vi "Main.vi"() -> ()   [LabVIEW 2012]
uses:
  MeasureDialogButton.ctl
  SourceDialogButton.ctl
  TriggerDialogButton.ctl
  DUTDisplayData.ctl
  DUTDialogButton.ctl
  LogDialogButton.ctl
  Setup.ctl
  DUTConfiguration.ctl
  driver/Public/Controls/SMUSense.ctl
  LogConfiguration.ctl
  LogStartConfiguration.ctl
  LogStartTriggerType.ctl
  LogDigitalIOTriggerEdge.ctl
  LogRolloverConfiguration.ctl
  LogRolloverTriggerType.ctl
  LogStopConfiguration.ctl
  LogStopTriggerType.ctl
  TriggerConfiguration.ctl
  TriggerInputConfiguration.ctl
  TriggerInputType.ctl
  driver/Public/Controls/TriggerMode.ctl
  TriggerOutputConfiguration.ctl
  TriggerOutputType.ctl
  SourceConfiguration.ctl
  SourceFunction.ctl
  MeasureConfiguration.ctl
  driver/Public/Controls/SMU.ctl
  UIActionQueueElement.ctl
  UIAction.ctl
  HardwareActionQueueElement.ctl
  HardwareAction.ctl
  HardwareAbortGlobalAction.ctl
  LogActionQueueElement.ctl
  LogAction.ctl
  driver/Keithley-2602.lvlib
  libs/LV-Utilities/LV-Utilities.lvlib
panel:
  in  "LIVE":bool
  in  "SYSTEM":bool
  out "Tab Control":enum32{"SYSTEM", "LIVE"}(tab)
  out "Digital IO Port":bool[](array[boolean])
  out "Setup File":path
  in  "RESET":bool
  in  "SAVE":bool
  in  "OPEN":bool
  in  "LOG START":bool
  out "Log Running?":bool
  in  "Hardware START":bool
  out "Hardware Running?":bool
  in  "SHOW LOG DIALOG":T1
  in  "SHOW DUT DIALOG":T2
  in  "SHOW SOURCE DIALOG":T3
  in  "SHOW TRIGGER DIALOG":T4
  in  "SHOW MEASURE DIALOG":T5
  out "System SMU B DUT Display Data":T6[](array[typedef]) {"Resistance (Ohm)" format="%_4p"; "Current (A)" format="%_4p"; "Voltage (V)" format="%_4p"}
  out "System SMU A DUT Display Data":T6[](array[typedef]) {"Resistance (Ohm)" format="%_4p"; "Current (A)" format="%_4p"; "Voltage (V)" format="%_4p"}
  out "Log File":path
  out "Live SMU Chart":dbl(graph)
  in  "Live Measure Value":enum16{"Voltage", "Current", "Resistance"}(ring)
  in  "Live SMU":enum16{"A", "B"}(ring)
  in  "Live DUT":u32=1 min=1 step=1
  out "Live SMU Value":dbl format="%_4p"
  out "Live SMU Units":enum16{"V", "A", "Ohm"}(ring)
  in  "CHART SMU DATA RESET":bool
  in  "DONE":bool
  # "DIGITAL IO"
  # "1"
  # "2"
  # "3"
  # "4"
  # "5"
  # "6"
  # "7"
  # "8"
  # "9"
  # "10"
  # "11"
  # "12"
  # "13"
  # "14"
  # "SETUP"
  # "LOG"
  # "RUN"
  # "SMU B"
  # "SMU A"
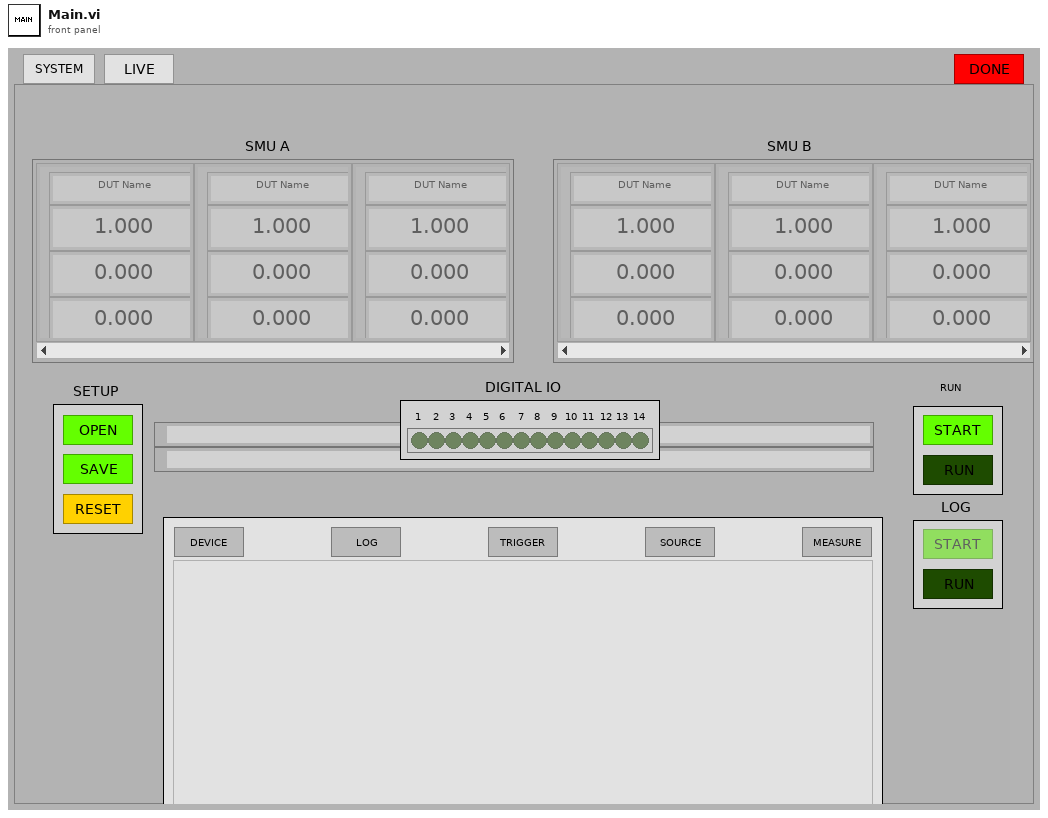
[diagram p1: front panel]
types:
  T1 = typedef "LogDialogButton.ctl" = bool
  T2 = typedef "DUTDialogButton.ctl" = bool
  T3 = typedef "SourceDialogButton.ctl" = bool
  T4 = typedef "TriggerDialogButton.ctl" = bool
  T5 = typedef "MeasureDialogButton.ctl" = bool
  T6 = typedef "DUTDisplayData.ctl" = cluster{"Name":string, "Voltage (V)":dbl, "Current (A)":dbl, "Resistance (Ohm)":dbl}
  T7 = typedef "Setup.ctl" = cluster{"DUT":T8, "Log":T10, "Trigger":T18, "Sources":T24[], "Measures":T26[]}
  T8 = typedef "DUTConfiguration.ctl" = cluster{"Count":u32, "Wirings":T9[], "Names":string[][]}
  T9 = typedef "Keithley-2602.lvlib/SMUSense.ctl" = enum16{"Local (2-wire)", "Remote (4-wire)", "Calibration"}
  T10 = typedef "LogConfiguration.ctl" = cluster{"Start":T11, "Rollover":T14, "Stop":T16}
  T11 = typedef "LogStartConfiguration.ctl" = cluster{"Trigger Type":T12, "Timer (sec)":dbl, "Digital IO Line":u8, "Digital IO Edge":T13}
  T12 = typedef "LogStartTriggerType.ctl" = enum16{"Immediate", "User", "Timer", "Digital IO"}
  T13 = typedef "LogDigitalIOTriggerEdge.ctl" = enum16{"Rising", "Falling"}
  T14 = typedef "LogRolloverConfiguration.ctl" = cluster{"Trigger Type":T15, "Timer (sec)":dbl, "File Size (MB)":u32, "Digital IO Line":u8, "Digital IO Edge":T13}
  T15 = typedef "LogRolloverTriggerType.ctl" = enum16{"None", "Timer", "File Size", "Digital IO"}
  T16 = typedef "LogStopConfiguration.ctl" = cluster{"Trigger Type":T17, "Timer (sec)":dbl, "File Size (MB)":u32, "Digital IO Line":u8, "Digital IO Edge":T13}
  T17 = typedef "LogStopTriggerType.ctl" = enum16{"None", "User", "Timer", "File Size", "Digital IO"}
  T18 = typedef "TriggerConfiguration.ctl" = cluster{"Input":T19, "Output":T22}
  T19 = typedef "TriggerInputConfiguration.ctl" = cluster{"Type":T20, "Timeout (ms)":u32, "Delay (ms)":u32, "Digital IO Line (1-14)":u8, "Digital IO Mode":T21}
  T20 = typedef "TriggerInputType.ctl" = enum16{"None", "Digital IO", "Bus"}
  T21 = typedef "Keithley-2602.lvlib/TriggerMode.ctl" = enum16{"Falling", "Rising", "Either", "Synchronous"}
  T22 = typedef "TriggerOutputConfiguration.ctl" = cluster{"Type":T23, "Delay (ms)":u32, "Digital IO Line (1-14)":u8, "Digital IO Mode":T21, "Digital IO Pulse Width (sec)":dbl}
  T23 = typedef "TriggerOutputType.ctl" = enum16{"None", "Digital IO", "Bus"}
  T24 = typedef "SourceConfiguration.ctl" = cluster{"Enabled?":bool, "Function":T25, "Level (V or A)":dbl, "Autorange Enabled?":bool, "High Limit (V or A)":dbl, "Low Limit (V or A)":dbl}
  T25 = typedef "SourceFunction.ctl" = enum16{"Voltage", "Current"}
  T26 = typedef "MeasureConfiguration.ctl" = cluster{"Enabled?":bool, "Count":u8, "Interval (sec)":dbl, "Voltage Auto Range Enabled?":bool, "Voltage High Limit (V or A)":dbl, "Voltage Low Limit (V or A)":dbl, "Current Auto Range Enabled?":bool, "Current High Limit (V or A)":dbl, "Current Low Limit (V or A)":dbl}
  T27 = typedef "ExecutableConfiguration.ctl" = cluster{"GPIB ID":u8, "GPIB Board":u8, "Default Data Folder":path, "Default Setup Folder":path}
  T28 = typedef "DataStructures.ctl" = cluster{"Display Data":refnum<notifier>, "Log Data":refnum<queue>}
  T29 = typedef "ActionQueues.ctl" = cluster{"UI Action":refnum<queue>, "Hardware Action":refnum<queue>, "Log Action":refnum<queue>}
  T30 = typedef "Keithley-2602.lvlib/SMU.ctl" = enum16{"A", "B"}
  T31 = enum8{"Enabled", "Disabled", "Disabled and Grayed Out"}
  T32 = typedef "UIActionQueueElement.ctl" = cluster{"Action":T33, "Data":variant}
  T33 = typedef "UIAction.ctl" = enum16{"Initialize", "Configure Trigger", "Configure Measure", "Configure Source", "Configure DUT", "Configure Log", "Configure Open", "Configure Save", "Configure Reset", "Hardware Start", "Hardware Started", "Hardware Stop", "Hardware Stopped", "Log Arm", "Log Start", "Log Started", "Log Stop", "Log Stopped", "Error", "Shutdown"}
  T34 = typedef "HardwareActionQueueElement.ctl" = cluster{"Action":T35, "Data":variant}
  T35 = typedef "HardwareAction.ctl" = enum16{"Initialize", "Start", "Run", "Stop", "Error", "Shutdown"}
  T36 = typedef "HardwareAbortGlobalAction.ctl" = enum16{"Set", "Get"}
  T37 = typedef "LogActionQueueElement.ctl" = cluster{"Action":T38, "Data":variant}
  T38 = typedef "LogAction.ctl" = enum16{"Initialize", "Start", "Arm", "Create", "Write", "Close", "Rearm", "Stop", "Error", "Shutdown"}
  T39 = typedef "HardwareDisplayData.ctl" = cluster{"DUT Names":string[][], "SMU":dbl[][], "Port":bool[]}
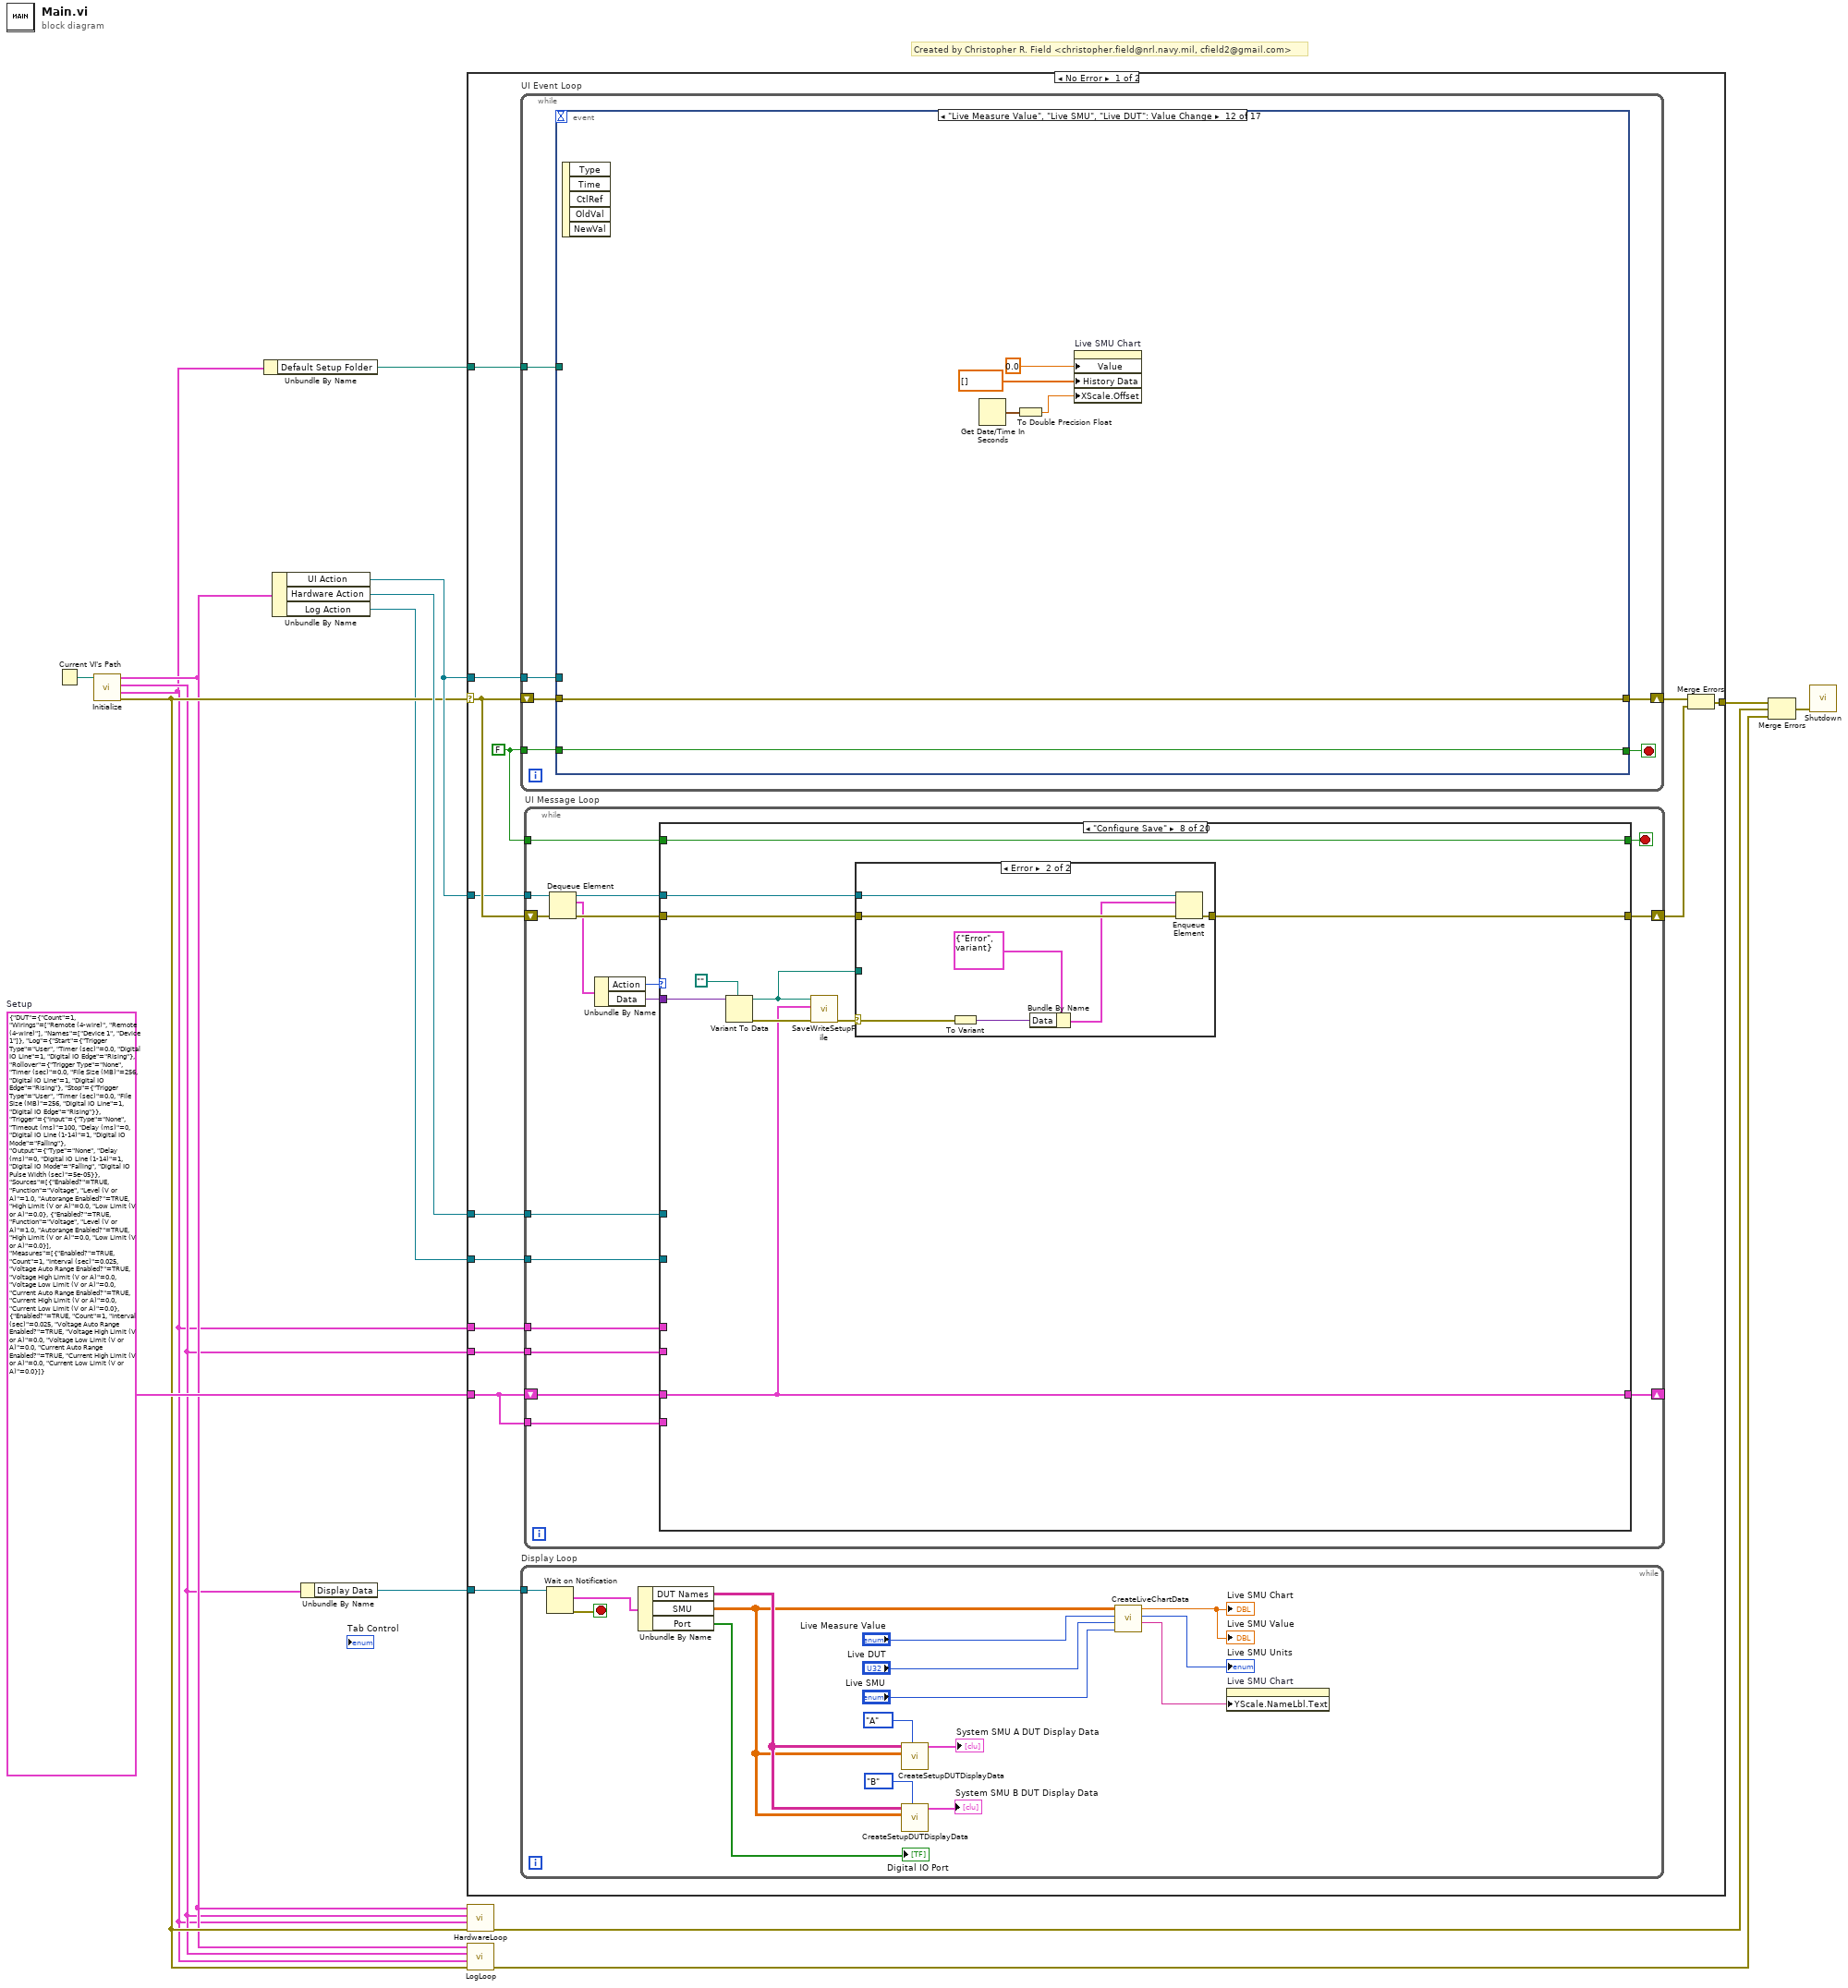
[diagram p0: block diagram]
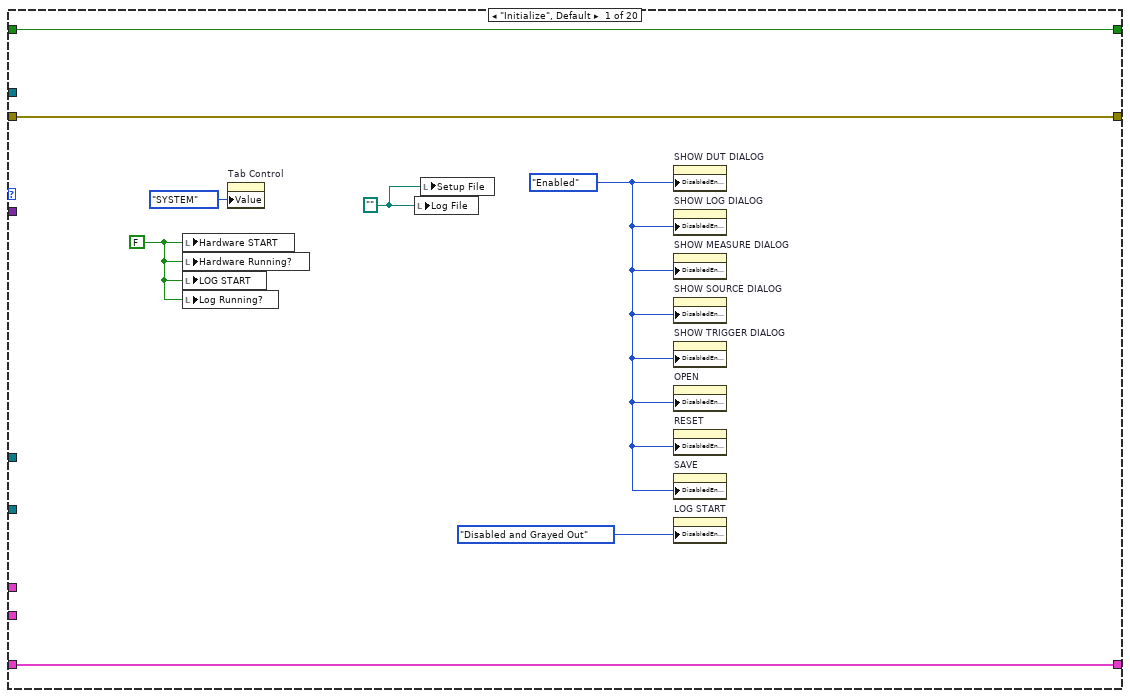
[diagram p2: hidden frame]
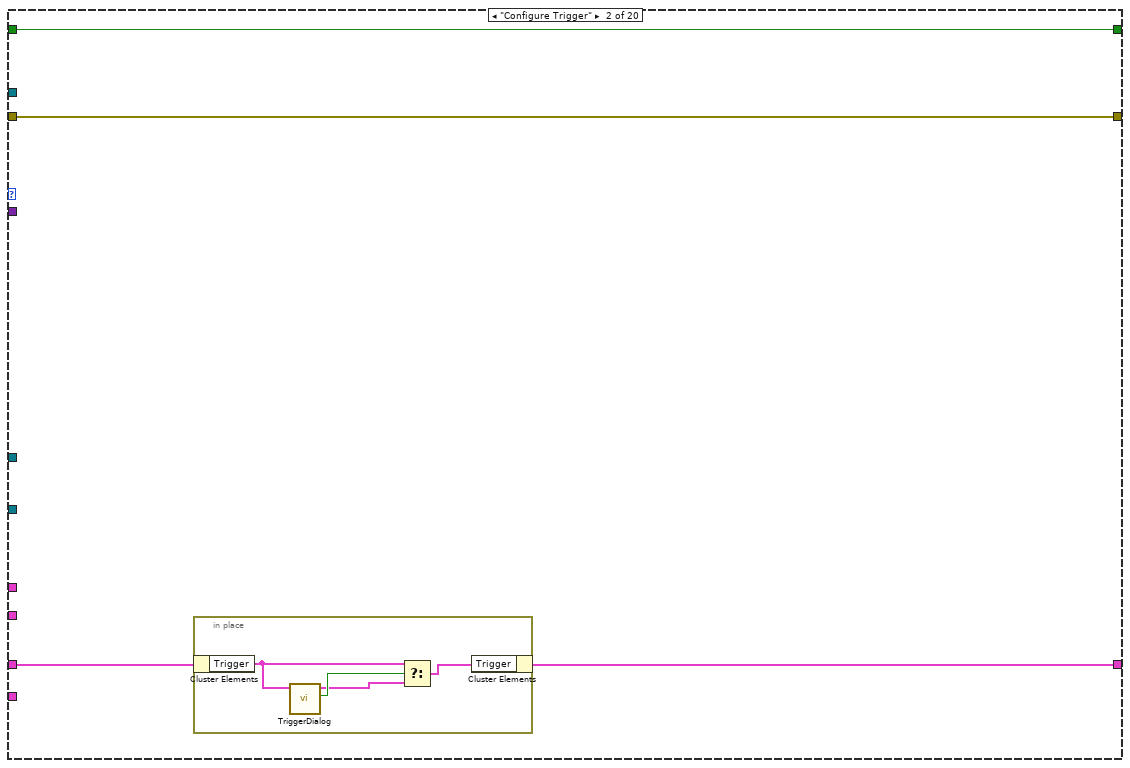
[diagram p3: hidden frame]
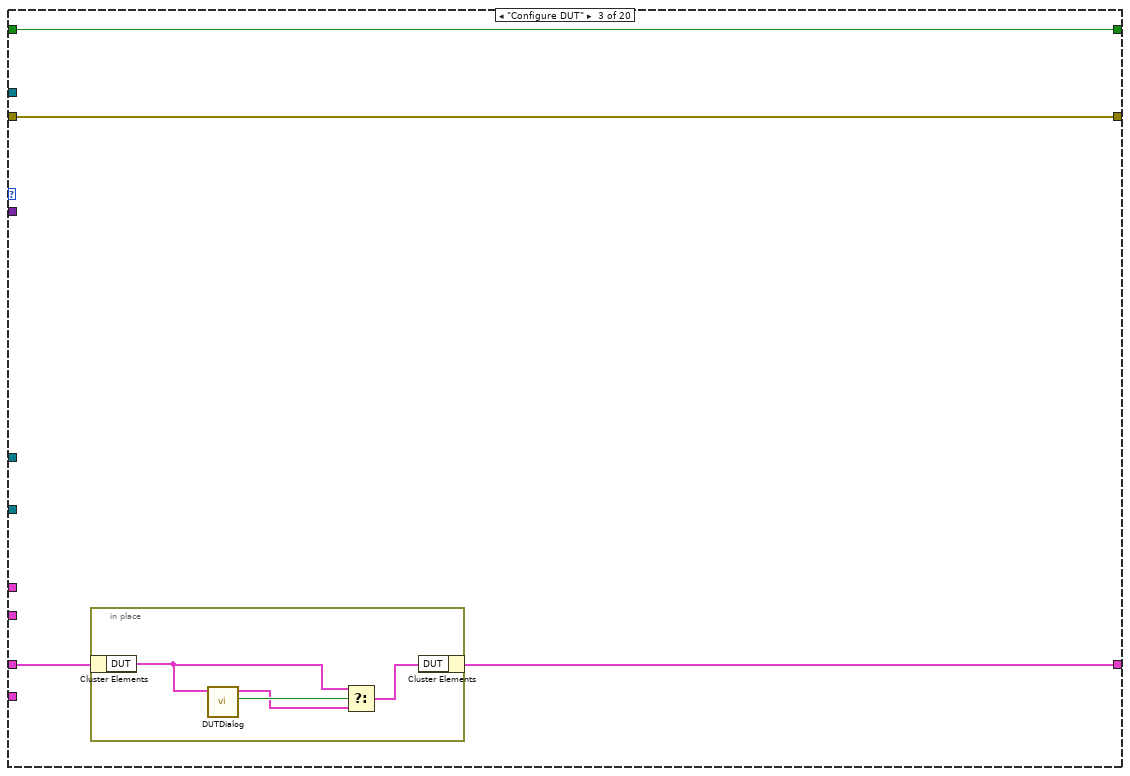
[diagram p4: hidden frame]
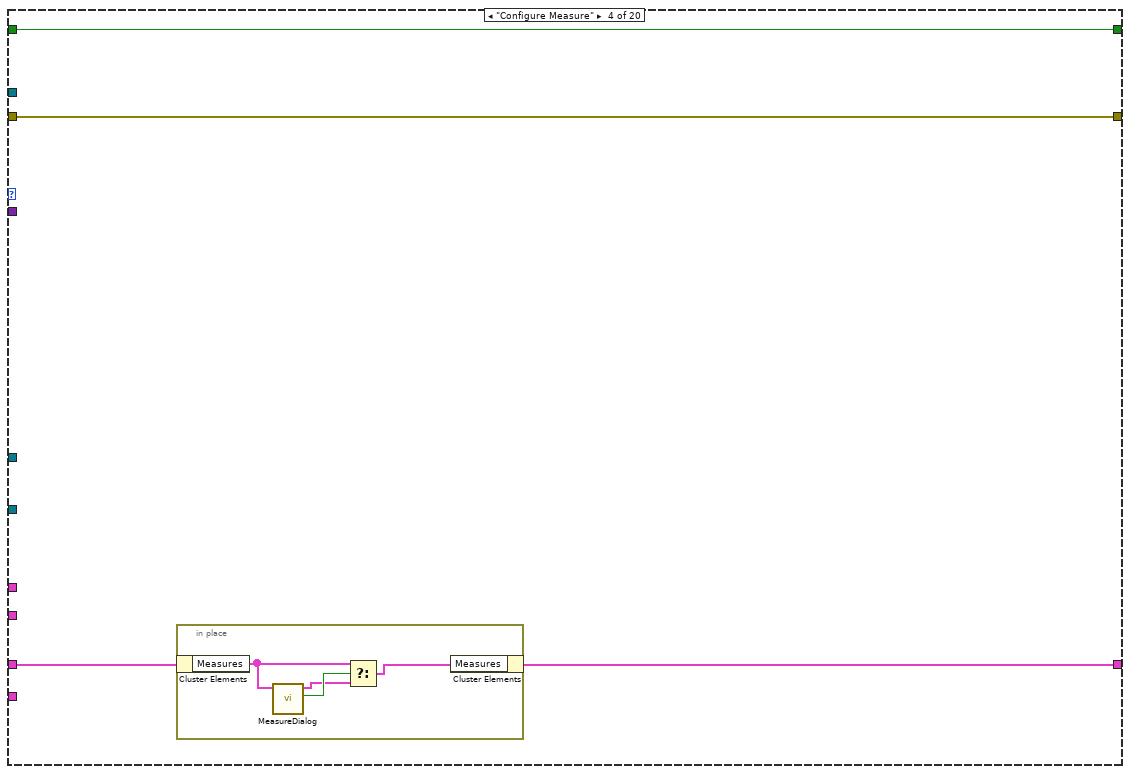
[diagram p5: hidden frame]
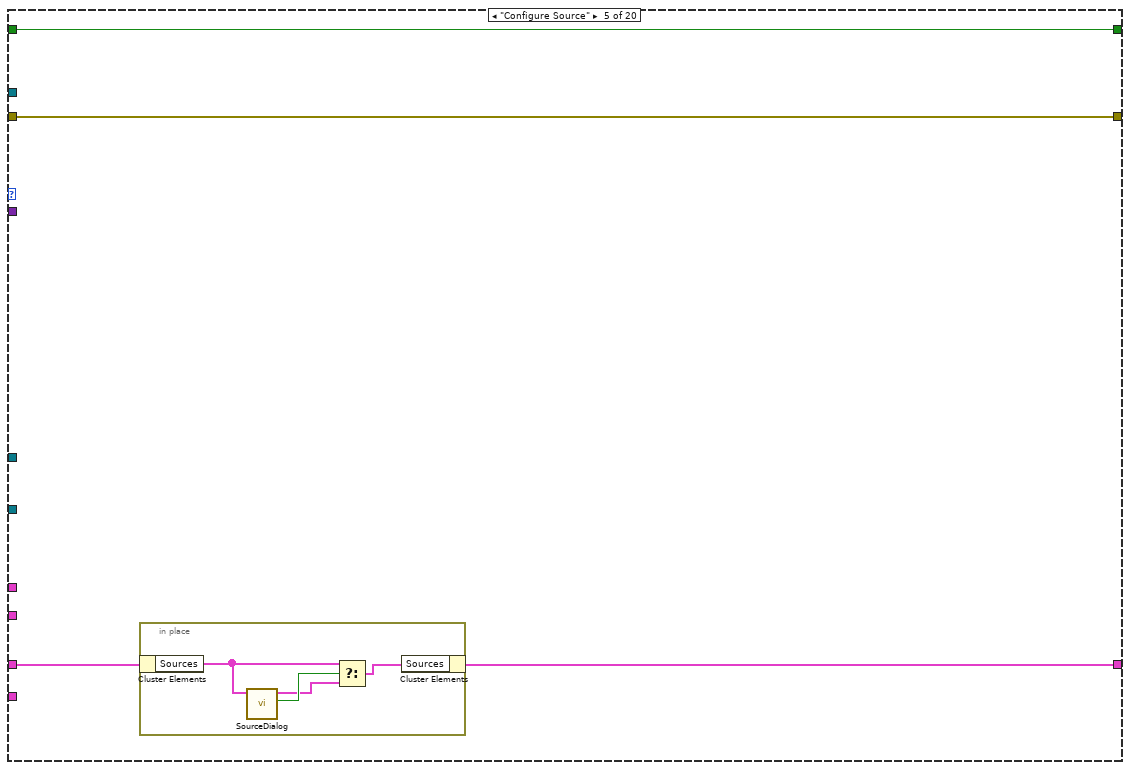
[diagram p6: hidden frame]
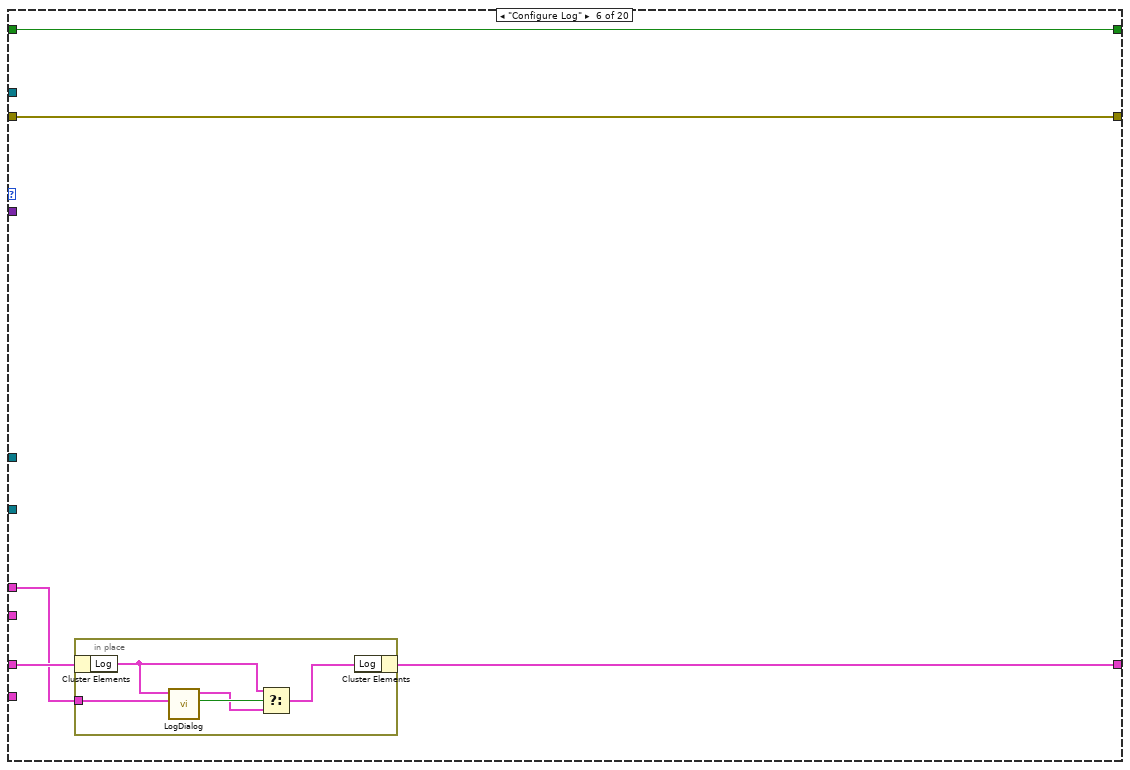
[diagram p7: hidden frame]
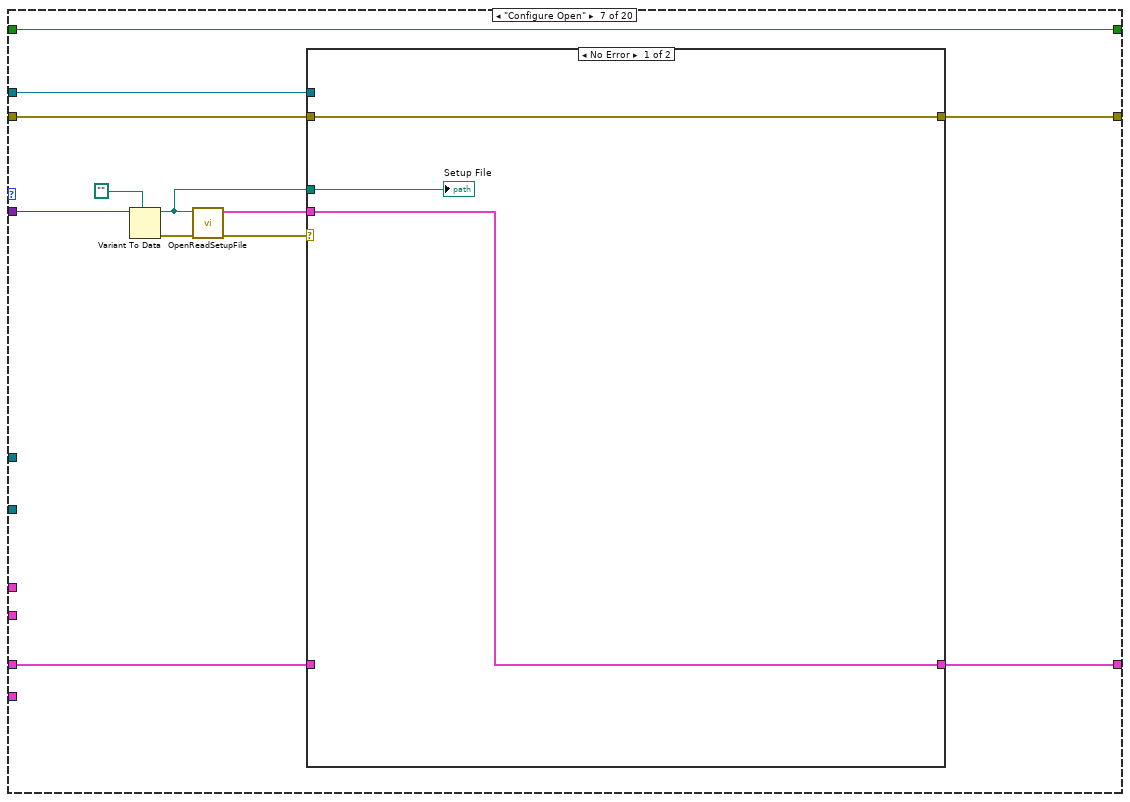
[diagram p8: hidden frame]
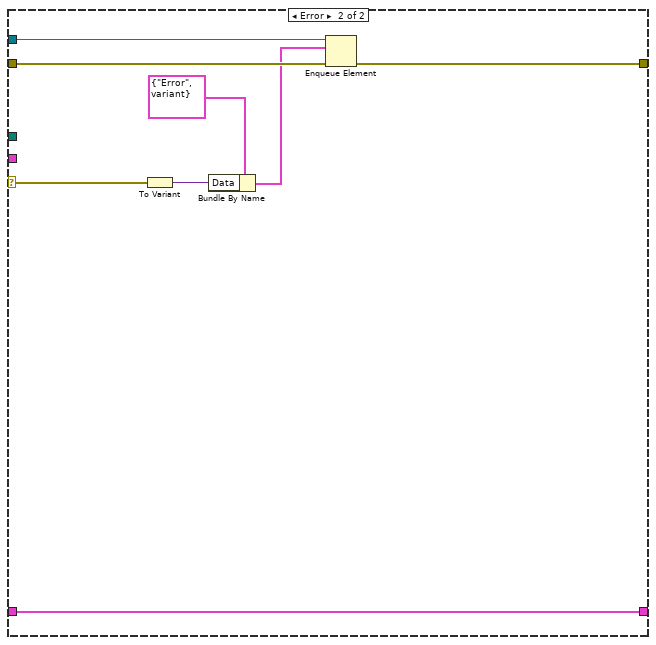
[diagram p9: hidden frame]
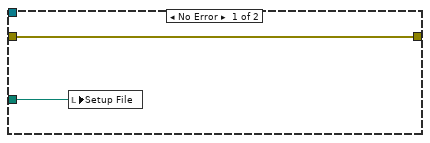
[diagram p10: hidden frame]
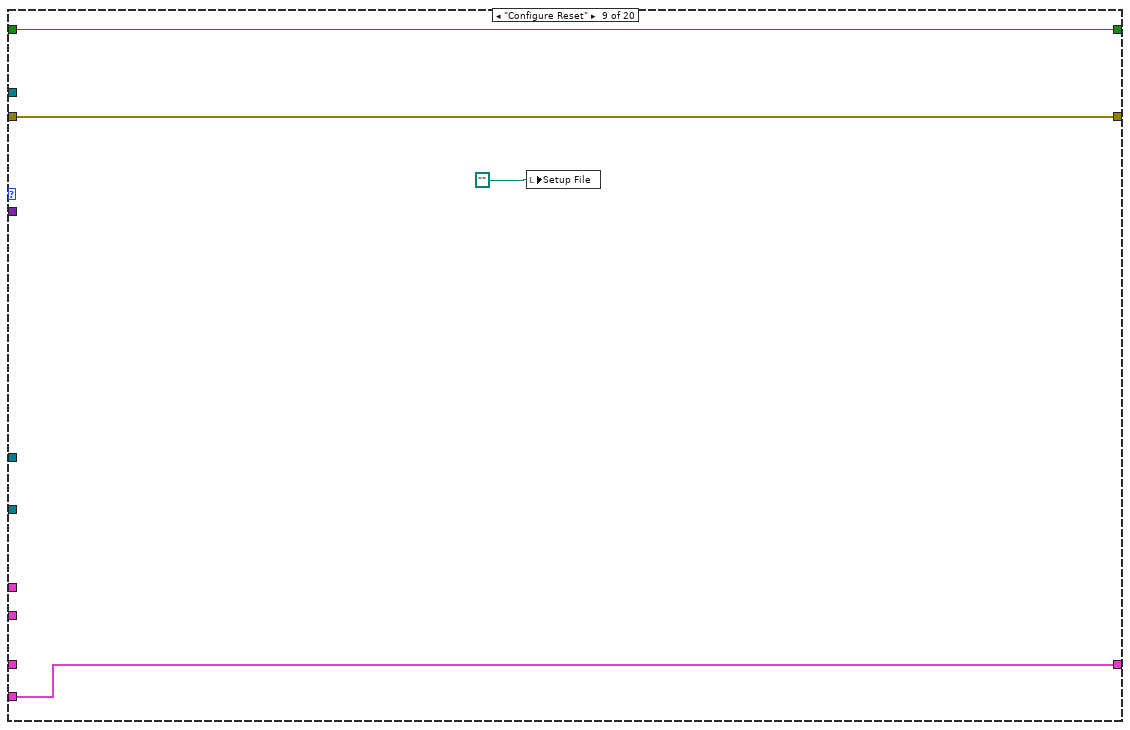
[diagram p11: hidden frame]
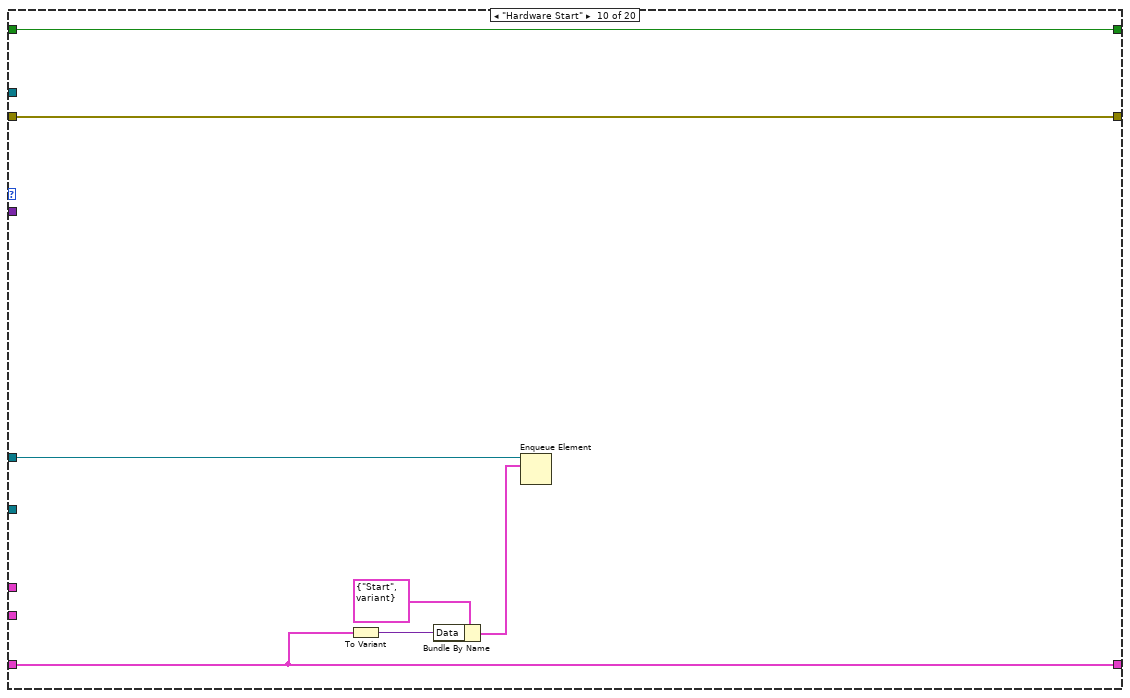
[diagram p12: hidden frame]
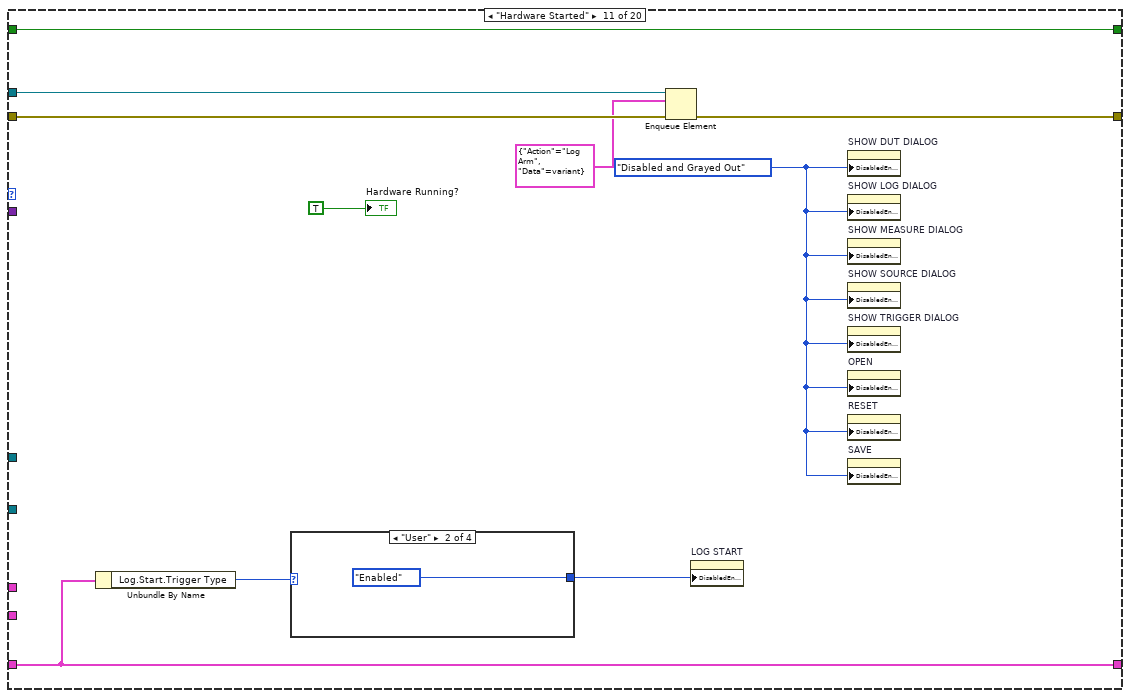
[diagram p13: hidden frame]
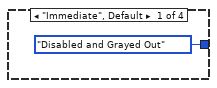
[diagram p14: hidden frame]
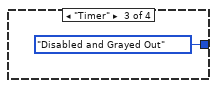
[diagram p15: hidden frame]
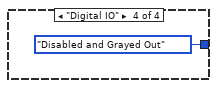
[diagram p16: hidden frame]
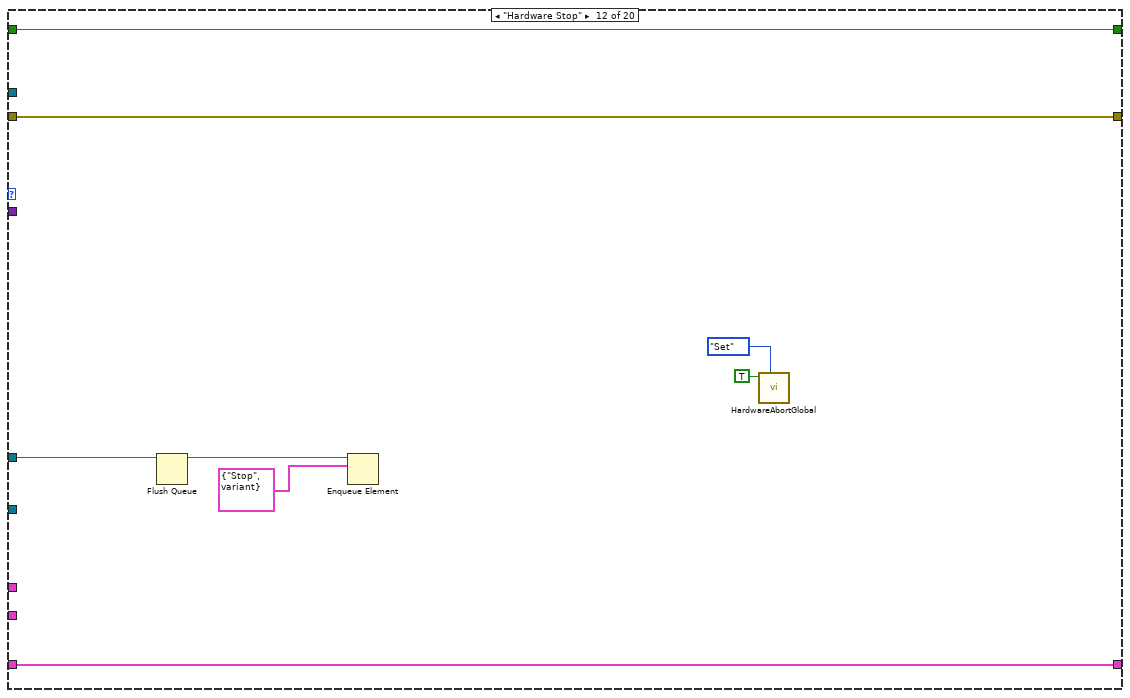
[diagram p17: hidden frame]
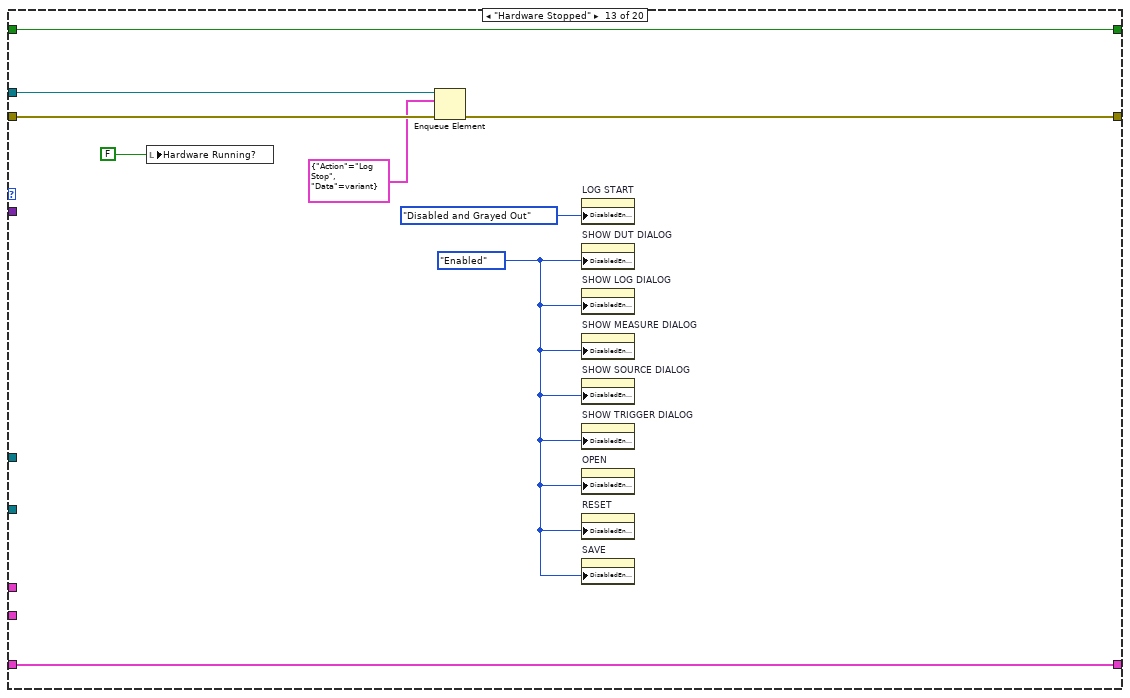
[diagram p18: hidden frame]
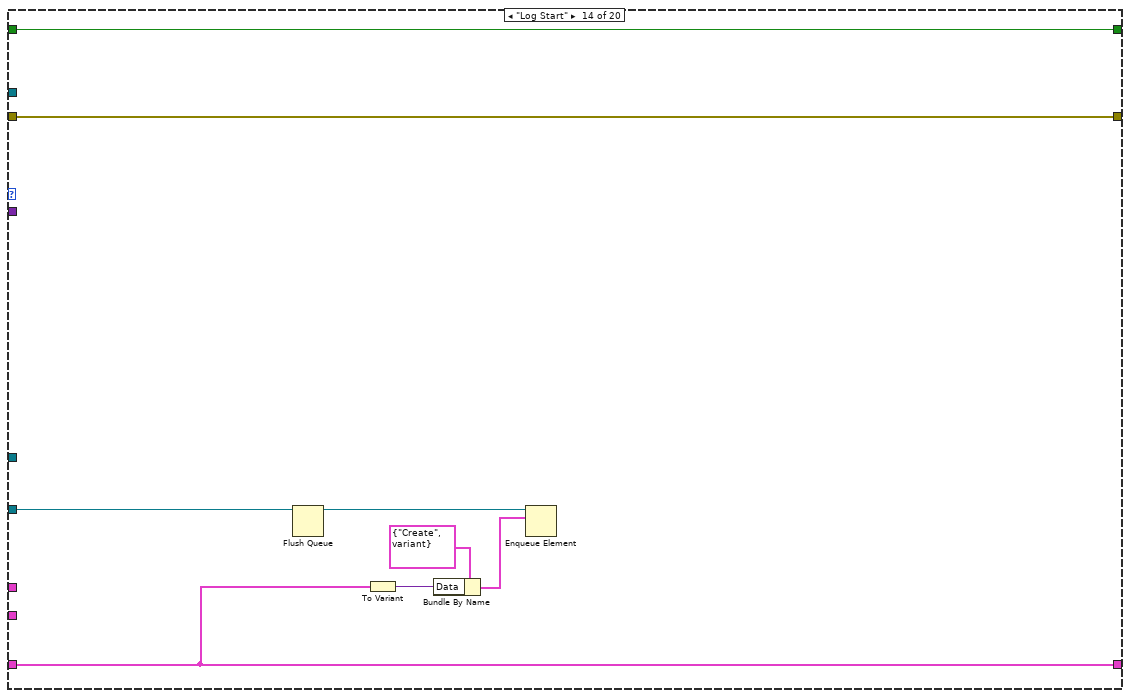
[diagram p19: hidden frame]
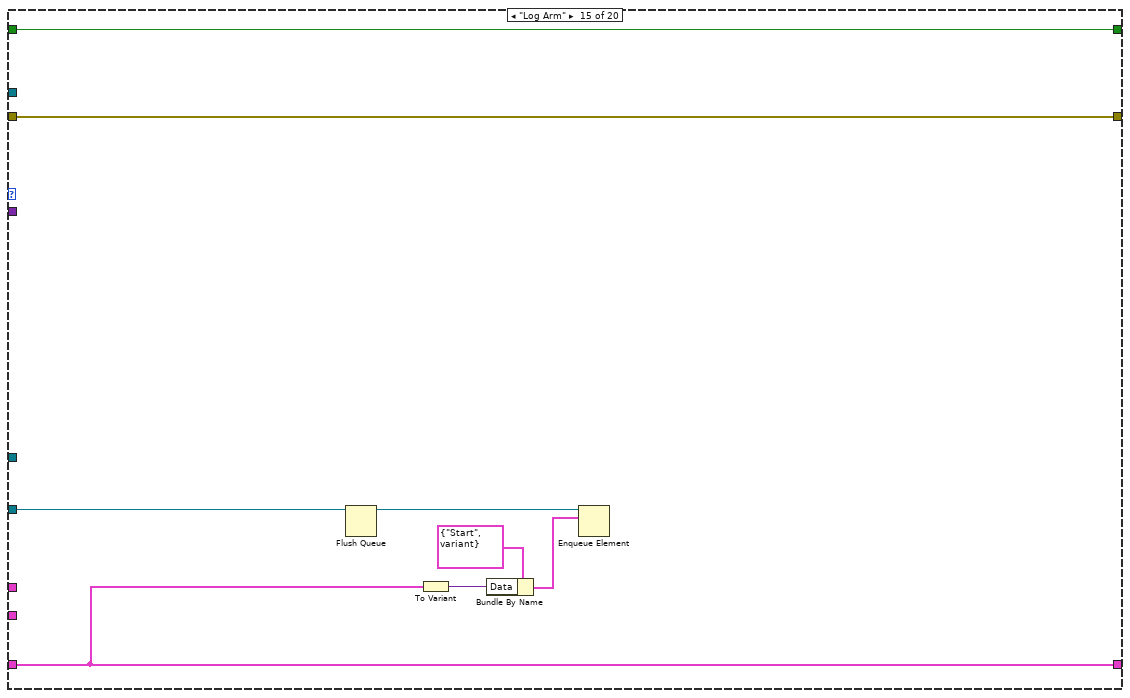
[diagram p20: hidden frame]
diagram:
  w9 = T7 {"DUT"={"Count"=1, "Wirings"=[enum."Remote (4-wire)", enum."Remote (4-wire)"], "Names"=[["Device 1"], ["Device 1"]]}, "Log"={"Start"={"Trigger Type"=enum."User", "Timer (sec)"=0.0, "Digital IO Line"=1, "Digital IO Edge"=enum."Rising"}, "Rollover"={"Trigger Type"=enum."None", "Timer (sec)"=0.0, "File Size (MB)"=256, "Digital IO Line"=1, "Digital IO Edge"=enum."Rising"}, "Stop"={"Trigger Type"=enum."User", "Timer (sec)"=0.0, "File Size (MB)"=256, "Digital IO Line"=1, "Digital IO Edge"=enum."Rising"}}, "Trigger"={"Input"={"Type"=enum."None", "Timeout (ms)"=100, "Delay (ms)"=0, "Digital IO Line (1-14)"=1, "Digital IO Mode"=enum."Falling"}, "Output"={"Type"=enum."None", "Delay (ms)"=0, "Digital IO Line (1-14)"=1, "Digital IO Mode"=enum."Falling", "Digital IO Pulse Width (sec)"=5e-05}}, "Sources"=[{"Enabled?"=TRUE, "Function"=enum."Voltage", "Level (V or A)"=1.0, "Autorange Enabled?"=TRUE, "High Limit (V or A)"=0.0, "Low Limit (V or A)"=0.0}, {"Enabled?"=TRUE, "Function"=enum."Voltage", "Level (V or A)"=1.0, "Autorange Enabled?"=TRUE, "High Limit (V or A)"=0.0, "Low Limit (V or A)"=0.0}], "Measures"=[{"Enabled?"=TRUE, "Count"=1, "Interval (sec)"=0.025, "Voltage Auto Range Enabled?"=TRUE, "Voltage High Limit (V or A)"=0.0, "Voltage Low Limit (V or A)"=0.0, "Current Auto Range Enabled?"=TRUE, "Current High Limit (V or A)"=0.0, "Current Low Limit (V or A)"=0.0}, {"Enabled?"=TRUE, "Count"=1, "Interval (sec)"=0.025, "Voltage Auto Range Enabled?"=TRUE, "Voltage High Limit (V or A)"=0.0, "Voltage Low Limit (V or A)"=0.0, "Current Auto Range Enabled?"=TRUE, "Current High Limit (V or A)"=0.0, "Current Low Limit (V or A)"=0.0}]}  # Setup
  # "Created by Christopher R. Field <christopher.field@nrl.navy.mil, cfield2@gmail.com>"
  n1 = Current VI's Path() -> (path=w10:path)
  n2 = call "Initialize.vi"("VI Path"=w10) -> ("Error Out"=w7:errorcluster, "Executable Configuration"=w2:T27, "Data Structures"=w5:T28, "Action Queues"=w6:T29)  [unwired: 7 in]
  n3 = Unbundle By Name(w2) -> ("Default Setup Folder"=w1:path)
  n4 = Unbundle By Name(w6) -> ("UI Action"=w15:refnum<queue>, "Hardware Action"=w11:refnum<queue>, "Log Action"=w3:refnum<queue>)
  n5 = Unbundle By Name(w5) -> ("Display Data"=w8:refnum<notifier>)
  n6 = case shown="No Error" w7 {
    selector: w7 -> [w27 w396]
    tunnel: [w28 w396] -> w14
    tunnel: w15 -> [w24 _]
    tunnel: w15 -> [w23 _]
    tunnel: w11 -> [w22 _]
    tunnel: w9 -> [w17 _]
    tunnel: w8 -> [w21 _]
    tunnel: w5 -> [w20 _]
    tunnel: w2 -> [w19 _]
    tunnel: w3 -> [w18 _]
    tunnel: w1 -> [w16 _]
    frame No Error {
      w25 = FALSE
      n7 = while "UI Event Loop" {
        tunnel: w25 -> [w277]
        shift-right: [w274] -> w29
        shift-left: w27 -> [w275]
        tunnel: w23 -> [w273]
        tunnel: w16 -> [w272]
        stop <- w276 stop-if-true
        n8 = event shown="[11] \"Live Measure Value\", \"Live SMU\", \"Live DUT\": Value Change" {
          selector: _ -> [_ _ _ _ _ _ _ _ _ _ _ _ _ _ _ _ _]
          dyn-events: _ -> [_ _ _ _ _ _ _ _ _ _ _ _ _ _ _ _ _]
          timeout: _ -> [_ _ _ _ _ _ _ _ _ _ _ _ _ _ _ _ _]
          tunnel: w277 -> [w279 w285 w290 w304 w320 w336 w341 w346 w348 w362 w367 w372 w375 w381 w387 w389 w394]
          tunnel: [w279 w284 w290 w304 w320 w336 w341 w346 w348 w361 w367 w372 w375 w381 w387 w389 w394] -> w276
          tunnel: w275 -> [w278 w281 w292 w295 w322 w334 w339 w344 w350 w357 w365 w373 w374 w382 w385 w391 w395]
          tunnel: [w278 w282 w291 w296 w321 w333 w338 w343 w349 w360 w364 w373 w374 w382 w384 w390 w395] -> w274
          tunnel: w273 -> [_ w283 w293 w297 w323 w335 w340 w345 w351 w358 w366 _ _ _ w386 w392 _]
          tunnel: w272 -> [_ _ _ w294 w313 _ _ _ _ _ _ _ _ _ _ _ _]
          event Timeout {
            n9 = event-data() -> ()  [unwired: 1 in, 2 out]
          }
          event Panel Close? {
            n10 = event-data() -> ()  [unwired: 1 in, 3 out]
            n11 = Not(x=w285) -> (.not. x?=w284:bool)
            n12 = Enqueue Element(queue=w283, element=T32 {"Action"=enum."Shutdown", "Data"=variant}, error in (no error)=w281) -> (error out=w282:errorcluster)  [unwired: 1 in, 2 out]
            n13 = event-data("Discard?"=w284) -> ()  [unwired: 1 in, 1 out]
          }
          event "LOG START": Value Change {
            n14 = event-data() -> ()  [unwired: 1 in, 5 out]
            n15 = Select(t=T32 {"Action"=enum."Log Start", "Data"=variant} ("element"), s="LOG START", f=T32 {"Action"=enum."Log Stop", "Data"=variant} ("element")) -> (s? t:f=w286:T32)
            n16 = Enqueue Element(queue=w293, element=w286, error in (no error)=w292) -> (error out=w291:errorcluster)  [unwired: 1 in, 2 out]
          }
          event "OPEN": Value Change {
            n17 = event-data() -> ()  [unwired: 1 in, 5 out]
            n18 = call "SelectFile.vi"("Button Label"="Open", "Prompt"="Select Setup File", "File Description"="Setup File", "File Extension (.*)"=".xml", "Start Path"=w294) -> ("Cancelled?"=w299:bool, "Selected File Path"=w298:path)  [unwired: 4 in, 1 out]
            n19 = case shown="False" w299 {
              tunnel: w297 -> [w311 _]
              tunnel: w295 -> [w310 w312]
              tunnel: [w309 w312] -> w296
              tunnel: w298 -> [w306 _]
              frame False {
                n20 = To Variant(anything=w306) -> (Variant=w307:variant)
                n21 = Bundle By Name(cluster=T32 {"Action"=enum."Configure Open", "Data"=variant} ("element"), "Data"=w307) -> (w305:T32)
                n22 = Enqueue Element(queue=w311, element=w305, error in (no error)=w310) -> (error out=w309:errorcluster)  [unwired: 1 in, 2 out]
              }
              frame True {
              }
            }
          }
          event "SAVE": Value Change {
            n23 = event-data() -> ()  [unwired: 1 in, 5 out]
            n24 = call "SelectFile.vi"("Button Label"="Save", "Prompt"="Select Setup File", "File Description"="Setup File", "File Extension (.*)"=".xml", "Start Path"=w313) -> ("Cancelled?"=w315:bool, "Selected File Path"=w314:path)  [unwired: 4 in, 1 out]
            n25 = case shown="False" w315 {
              tunnel: w323 -> [w330 _]
              tunnel: w322 -> [w329 w331]
              tunnel: [w328 w331] -> w321
              tunnel: w314 -> [w325 _]
              frame False {
                n26 = To Variant(anything=w325) -> (Variant=w326:variant)
                n27 = Bundle By Name(cluster=T32 {"Action"=enum."Configure Save", "Data"=variant} ("element"), "Data"=w326) -> (w324:T32)
                n28 = Enqueue Element(queue=w330, element=w324, error in (no error)=w329) -> (error out=w328:errorcluster)  [unwired: 1 in, 2 out]
              }
              frame True {
              }
            }
          }
          event "RESET": Value Change {
            n29 = event-data() -> ()  [unwired: 1 in, 5 out]
            n30 = Enqueue Element(queue=w335, element=T32 {"Action"=enum."Configure Reset", "Data"=variant}, error in (no error)=w334) -> (error out=w333:errorcluster)  [unwired: 1 in, 2 out]
          }
          event Value Change {
            n31 = event-data() -> ()  [unwired: 1 in, 1 out]
            n32 = Enqueue Element(queue=w340, element=T32 {"Action"=enum."Configure Measure", "Data"=variant}, error in (no error)=w339) -> (error out=w338:errorcluster)  [unwired: 1 in, 2 out]
          }
          event Value Change {
            n33 = event-data() -> ()  [unwired: 1 in, 5 out]
            n34 = Enqueue Element(queue=w345, element=T32 {"Action"=enum."Configure Source", "Data"=variant}, error in (no error)=w344) -> (error out=w343:errorcluster)  [unwired: 1 in, 2 out]
          }
          event "Hardware START": Value Change {
            n35 = event-data() -> ()  [unwired: 1 in, 1 out]
            n36 = Select(t=T32 {"Action"=enum."Hardware Start", "Data"=variant} ("UI Action Queue Element"), s="Hardware START", f=T32 {"Action"=enum."Hardware Stop", "Data"=variant} ("UI Action Queue Element")) -> (s? t:f=w347:T32)
            n37 = Enqueue Element(queue=w351, element=w347, error in (no error)=w350) -> (error out=w349:errorcluster)  [unwired: 1 in, 2 out]
          }
          event "DONE": Value Change {
            n38 = event-data() -> ()  [unwired: 1 in, 5 out]
            n39 = Not(x=w362) -> (.not. x?=w361:bool)
            n40 = Flush Queue(queue=w358, error in (no error)=w357) -> (queue out=w355:refnum<queue>, error out=w356:errorcluster)  [unwired: 1 out]
            n41 = Enqueue Element(queue=w355, element=T32 {"Action"=enum."Shutdown", "Data"=variant}, error in (no error)=w356) -> (error out=w360:errorcluster)  [unwired: 1 in, 2 out]
          }
          event Value Change {
            n42 = event-data() -> ()  [unwired: 1 in, 5 out]
            n43 = Enqueue Element(queue=w366, element=T32 {"Action"=enum."Configure Trigger", "Data"=variant}, error in (no error)=w365) -> (error out=w364:errorcluster)  [unwired: 1 in, 2 out]
          }
          event "Live Measure Value", "Live SMU", "Live DUT": Value Change {
            n44 = event-data() -> ()  [unwired: 1 in, 5 out]
            n45 = Get Date/Time In Seconds() -> (seconds since 1Jan1904=w369:timestamp)
            n46 = To Double Precision Float(number=w369) -> (double precision float=w368:dbl)
            n47 = property on="Live SMU Chart" class="WFChart (strict)"("Value"=0.0 ("Chart"), "History Data"=dbl[] [], "XScale.Offset"=w368) -> ()  [unwired: 2 in, 2 out]
          }
          event "CHART SMU DATA RESET": Value Change {
            n48 = event-data() -> ()  [unwired: 1 in, 5 out]
            n49 = Get Date/Time In Seconds() -> (seconds since 1Jan1904=w377:timestamp)
            n50 = To Double Precision Float(number=w377) -> (double precision float=w376:dbl)
            n51 = property on="Live SMU Chart" class="WFChart (strict)"("Value"=0.0 ("Chart"), "History Data"=dbl[] [], "XScale.Offset"=w376) -> ()  [unwired: 2 in, 2 out]
          }
          event "SYSTEM": Value Change {
            n52 = event-data() -> ()  [unwired: 1 in, 5 out]
            n53 = property on="Tab Control" class="TabCtl (strict)"("Value"=enum32{"SYSTEM", "LIVE"}."SYSTEM" ("Tab Control")) -> ()  [unwired: 2 in, 2 out]
          }
          event Value Change {
            n54 = event-data() -> ()  [unwired: 1 in, 5 out]
            n55 = Enqueue Element(queue=w386, element=T32 {"Action"=enum."Configure DUT", "Data"=variant}, error in (no error)=w385) -> (error out=w384:errorcluster)  [unwired: 1 in, 2 out]
          }
          event Value Change {
            n56 = event-data() -> ()  [unwired: 1 in, 5 out]
            n57 = Enqueue Element(queue=w392, element=T32 {"Action"=enum."Configure Log", "Data"=variant}, error in (no error)=w391) -> (error out=w390:errorcluster)  [unwired: 1 in, 2 out]
          }
          event "LIVE": Value Change {
            n58 = event-data() -> ()  [unwired: 1 in, 5 out]
            n59 = property on="Tab Control" class="TabCtl (strict)"("Value"=enum32{"SYSTEM", "LIVE"}."LIVE" ("Tab Control")) -> ()  [unwired: 2 in, 2 out]
          }
        }
      }
      n60 = while "Display Loop" {
        tunnel: w21 -> [w45]
        stop <- w44 stop-if-true
        n61 = Wait on Notification(notifier=w45) -> (notification=w43:T39, error out=w44:errorcluster)  [unwired: 3 in, 2 out]
        n62 = Unbundle By Name(w43) -> ("DUT Names"=w39:string[][], "SMU"=w36:dbl[][], "Port"=→"Digital IO Port":bool[])
        n63 = call "CreateSetupDUTDisplayData.vi"("SMU"=SMU."A", "SMU Data"=w36, "DUT Names"=w39) -> ("DUT Display Data"=→"System SMU A DUT Display Data":T6[])  [unwired: 8 in]
        n64 = call "CreateSetupDUTDisplayData.vi"("SMU"=SMU."B", "SMU Data"=w36, "DUT Names"=w39) -> ("DUT Display Data"=→"System SMU B DUT Display Data":T6[])  [unwired: 8 in]
        n65 = call "CreateLiveChartData.vi"("Live SMU"="Live SMU", "Live DUT"="Live DUT", "Live Measure Value"="Live Measure Value", "SMU"=w36) -> ("Live SMU Chart Y Scale Name"=w33:string, "Live SMU Units"=→"Live SMU Units":enum16{"V", "A", "Ohm"}, "Live SMU Chart"=→"Live SMU Chart" →"Live SMU Value":dbl)  [unwired: 5 in]
        n66 = property on="Live SMU Chart" class="WFChart (strict)"("YScale.NameLbl.Text"=w33) -> ()  [unwired: 2 in, 2 out]
      }
      n67 = while "UI Message Loop" {
        shift-right: [w61] -> w26
        shift-left: w27 -> [w59]
        tunnel: w25 -> [w62]
        tunnel: w24 -> [w58]
        tunnel: w22 -> [w52]
        shift-right: [w50] -> _
        shift-left: w17 -> [w51]
        tunnel: w20 -> [w49]
        tunnel: w19 -> [w48]
        tunnel: w18 -> [w47]
        tunnel: w17 -> [w46]
        stop <- w60 stop-if-true
        n68 = Dequeue Element(queue=w58, error in (no error)=w59) -> (queue out=w56:refnum<queue>, element=w55:T32, error out=w57:errorcluster)  [unwired: 1 in, 1 out]
        n69 = Unbundle By Name(w55) -> ("Action"=w54:T33, "Data"=w53:variant)
        n70 = case shown="\"Configure Save\"" w54 {
          tunnel: w62 -> [w70 w74 w82 w90 w98 w107 w124 w145 w158 w165 w175 w187 w196 w204 w212 w221 w233 w240 w253 w267]
          tunnel: w57 -> [w69 w73 w81 w89 w97 w106 w114 w137 w157 w164 w169 w186 w192 w203 w205 w220 w232 w241 w250 w264]
          tunnel: [w69 w73 w81 w89 w97 w106 w113 w136 w157 w164 w168 w186 w191 w203 w205 w220 w232 w241 w250 w263] -> w61
          tunnel: [w70 w74 w82 w90 w98 w107 w124 w145 w158 w165 w175 w187 w196 w204 w212 w221 w233 w240 w253 w266] -> w60
          tunnel: w56 -> [_ _ _ _ _ _ w115 w138 _ _ w170 _ w193 _ _ _ _ _ _ w265]
          tunnel: w53 -> [_ _ _ _ _ _ w123 w143 _ _ _ _ _ _ _ w219 _ _ w251 _]
          tunnel: w52 -> [_ _ _ _ _ _ _ _ _ w163 _ w183 _ _ _ _ _ _ _ w262]
          tunnel: w51 -> [w68 w72 w80 w88 w96 w105 w117 w141 _ w160 w173 w185 w194 w197 w206 w214 w231 w237 w252 w260]
          tunnel: [w68 w71 w79 w87 w95 w104 w118 w141 w156 w160 w173 w185 w194 w197 w206 w214 w231 w237 w252 w260] -> w50
          tunnel: w49 -> [_ _ _ _ _ _ _ _ _ _ _ _ _ _ _ _ _ _ _ _]
          tunnel: w48 -> [_ _ _ _ _ w103 _ _ _ _ _ _ _ _ _ _ _ _ _ _]
          tunnel: w47 -> [_ _ _ _ _ _ _ _ _ _ _ _ _ w199 w207 _ w230 _ _ w259]
          tunnel: w46 -> [_ _ _ _ _ _ _ _ w156 _ _ _ _ _ _ _ _ _ _ _]
          frame "Initialize", Default {
            w63 = T31."Enabled" ("Disabled")
            w64 = path ""
            w66 = FALSE ("START")
            n71 = local write "Hardware START"(w66) -> ()
            n72 = local write "Hardware Running?"(w66) -> ()
            n73 = local write "LOG START"(w66) -> ()
            n74 = local write "Log Running?"(w66) -> ()
            n75 = property on="Tab Control" class="TabCtl (strict)"("Value"=enum32{"SYSTEM", "LIVE"}."SYSTEM" ("Tab Control")) -> ()  [unwired: 2 in, 2 out]
            n76 = local write "Log File"(w64) -> ()
            n77 = local write "Setup File"(w64) -> ()
            n78 = property on="SHOW DUT DIALOG" class="Bool"("DisabledEnum"=w63) -> ()  [unwired: 2 in, 2 out]
            n79 = property on="SHOW LOG DIALOG" class="Bool"("DisabledEnum"=w63) -> ()  [unwired: 2 in, 2 out]
            n80 = property on="SHOW MEASURE DIALOG" class="Bool"("DisabledEnum"=w63) -> ()  [unwired: 2 in, 2 out]
            n81 = property on="SHOW SOURCE DIALOG" class="Bool"("DisabledEnum"=w63) -> ()  [unwired: 2 in, 2 out]
            n82 = property on="SHOW TRIGGER DIALOG" class="Bool"("DisabledEnum"=w63) -> ()  [unwired: 2 in, 2 out]
            n83 = property on="OPEN" class="Bool"("DisabledEnum"=w63) -> ()  [unwired: 2 in, 2 out]
            n84 = property on="RESET" class="Bool"("DisabledEnum"=w63) -> ()  [unwired: 2 in, 2 out]
            n85 = property on="SAVE" class="Bool"("DisabledEnum"=w63) -> ()  [unwired: 2 in, 2 out]
            n86 = property on="LOG START" class="Bool (strict)"("DisabledEnum"=T31."Disabled and Grayed Out" ("Disabled")) -> ()  [unwired: 2 in, 2 out]
          }
          frame "Configure Trigger" {
            n87 = in-place {
              n88 = in-place-cluster #1(w72) -> ("Trigger"=w77:T18)
              n89 = call "TriggerDialog.vi"("Trigger Configuration In"=w77) -> ("Cancelled"=w78:bool, "Trigger Configuration Out"=w76:T18)  [unwired: 8 in, 1 out]
              n90 = Select(t=w77, s=w78, f=w76) -> (s? t:f=w75:T18)
              n91 = in-place-cluster #1("Trigger"=w75) -> (w71:T7)
            }
          }
          frame "Configure DUT" {
            n92 = in-place {
              n93 = in-place-cluster #2(w80) -> ("DUT"=w85:T8)
              n94 = call "DUTDialog.vi"("DUT Configuration In"=w85) -> ("Cancelled?"=w86:bool, "DUT Configuration Out"=w84:T8)  [unwired: 8 in, 1 out]
              n95 = Select(t=w85, s=w86, f=w84) -> (s? t:f=w83:T8)
              n96 = in-place-cluster #2("DUT"=w83) -> (w79:T7)
            }
          }
          frame "Configure Measure" {
            n97 = in-place {
              n98 = in-place-cluster #3(w88) -> ("Measures"=w93:T26[])
              n99 = call "MeasureDialog.vi"("Measure Configuration In"=w93) -> ("Cancelled?"=w94:bool, "Measure Configuration Out"=w91:T26[])  [unwired: 8 in, 1 out]
              n100 = Select(t=w93, s=w94, f=w91) -> (s? t:f=w92:T26[])
              n101 = in-place-cluster #3("Measures"=w92) -> (w87:T7)
            }
          }
          frame "Configure Source" {
            n102 = in-place {
              n103 = in-place-cluster #4(w96) -> ("Sources"=w102:T24[])
              n104 = call "SourceDialog.vi"("Source Configurations In"=w102) -> ("Cancelled?"=w101:bool, "Source Configurations Out"=w100:T24[])  [unwired: 8 in, 1 out]
              n105 = Select(t=w102, s=w101, f=w100) -> (s? t:f=w99:T24[])
              n106 = in-place-cluster #4("Sources"=w99) -> (w95:T7)
            }
          }
          frame "Configure Log" {
            n107 = in-place {
              in-place-border: w103 -> [w108]
              n108 = in-place-cluster #5(w105) -> ("Log"=w109:T10)
              n109 = call "LogDialog.vi"("Executable Configuration"=w108, "Log Configuration In"=w109) -> ("Cancelled?"=w112:bool, "Log Configuration Out"=w111:T10)  [unwired: 7 in, 1 out]
              n110 = Select(t=w109, s=w112, f=w111) -> (s? t:f=w110:T10)
              n111 = in-place-cluster #5("Log"=w110) -> (w104:T7)
            }
          }
          frame "Configure Open" {
            n112 = Variant To Data(type=path "", Variant=w123) -> (data=w116:path, error out=w121:errorcluster)  [unwired: 1 in]
            n113 = call "OpenReadSetupFile.vi"("Error In"=w121, "Setup File"=w116) -> ("Error Out"=w120:errorcluster, "Setup"=w119:T7)  [unwired: 8 in]
            n114 = case shown="No Error" w120 {
              selector: w120 -> [_ w129]
              tunnel: w119 -> [w127 _]
              tunnel: [w127 w135] -> w118
              tunnel: w117 -> [_ w135]
              tunnel: w116 -> [w126 _]
              tunnel: w115 -> [_ w134]
              tunnel: w114 -> [w125 w133]
              tunnel: [w125 w132] -> w113
              frame No Error {
                "Setup File" <- w126
              }
              frame Error {
                n115 = To Variant(anything=w129) -> (Variant=w130:variant)
                n116 = Bundle By Name(cluster=T32 {"Action"=enum."Error", "Data"=variant} ("element"), "Data"=w130) -> (w128:T32)
                n117 = Enqueue Element(queue=w134, element=w128, error in (no error)=w133) -> (error out=w132:errorcluster)  [unwired: 1 in, 2 out]
              }
            }
          }
          frame "Configure Save" {
            n118 = Variant To Data(type=path "", Variant=w143) -> (data=w140:path, error out=w142:errorcluster)  [unwired: 1 in]
            n119 = call "SaveWriteSetupFile.vi"("Error In"=w142, "Setup"=w141, "Save File"=w140) -> ("Error Out"=w139:errorcluster)  [unwired: 8 in]
            n120 = case shown="Error" w139 {
              selector: w139 -> [_ w149]
              tunnel: w140 -> [w147 _]
              tunnel: w138 -> [_ w154]
              tunnel: w137 -> [w146 w153]
              tunnel: [w146 w152] -> w136
              frame No Error {
                n121 = local write "Setup File"(w147) -> ()
              }
              frame Error {
                n122 = To Variant(anything=w149) -> (Variant=w150:variant)
                n123 = Bundle By Name(cluster=T32 {"Action"=enum."Error", "Data"=variant} ("element"), "Data"=w150) -> (w148:T32)
                n124 = Enqueue Element(queue=w154, element=w148, error in (no error)=w153) -> (error out=w152:errorcluster)  [unwired: 1 in, 2 out]
              }
            }
          }
          frame "Configure Reset" {
            n125 = local write "Setup File"(path "") -> ()
          }
          frame "Hardware Start" {
            n126 = To Variant(anything=w160) -> (Variant=w161:variant)
            n127 = Bundle By Name(cluster=T34 {"Action"=enum."Start", "Data"=variant} ("element"), "Data"=w161) -> (w159:T34)
            n128 = Enqueue Element(queue=w163, element=w159) -> ()  [unwired: 2 in, 3 out]
          }
          frame "Hardware Started" {
            w166 = T31."Disabled and Grayed Out" ("Disabled")
            n129 = Unbundle By Name(w173) -> ("Log.Start.Trigger Type"=w172:T12)
            n130 = case shown="\"User\"" w172 {
              tunnel: [T31."Disabled and Grayed Out" ("Disabled") T31."Enabled" ("Disabled") T31."Disabled and Grayed Out" ("Disabled") T31."Disabled and Grayed Out" ("Disabled")] -> w171
              frame "Immediate", Default {
              }
              frame "User" {
              }
              frame "Timer" {
              }
              frame "Digital IO" {
              }
            }
            n131 = Enqueue Element(queue=w170, element=T32 {"Action"=enum."Log Arm", "Data"=variant}, error in (no error)=w169) -> (error out=w168:errorcluster)  [unwired: 1 in, 2 out]
            n132 = property on="LOG START" class="Bool (strict)"("DisabledEnum"=w171) -> ()  [unwired: 2 in, 2 out]
            n133 = property on="SHOW DUT DIALOG" class="Bool"("DisabledEnum"=w166) -> ()  [unwired: 2 in, 2 out]
            n134 = property on="SHOW LOG DIALOG" class="Bool"("DisabledEnum"=w166) -> ()  [unwired: 2 in, 2 out]
            n135 = property on="SHOW MEASURE DIALOG" class="Bool"("DisabledEnum"=w166) -> ()  [unwired: 2 in, 2 out]
            n136 = property on="SHOW SOURCE DIALOG" class="Bool"("DisabledEnum"=w166) -> ()  [unwired: 2 in, 2 out]
            n137 = property on="SHOW TRIGGER DIALOG" class="Bool"("DisabledEnum"=w166) -> ()  [unwired: 2 in, 2 out]
            n138 = property on="OPEN" class="Bool"("DisabledEnum"=w166) -> ()  [unwired: 2 in, 2 out]
            n139 = property on="RESET" class="Bool"("DisabledEnum"=w166) -> ()  [unwired: 2 in, 2 out]
            n140 = property on="SAVE" class="Bool"("DisabledEnum"=w166) -> ()  [unwired: 2 in, 2 out]
            "Hardware Running?" <- TRUE ("Run Running?")
          }
          frame "Hardware Stop" {
            n141 = Flush Queue(queue=w183) -> (queue out=w182:refnum<queue>)  [unwired: 1 in, 2 out]
            n142 = Enqueue Element(queue=w182, element=T34 {"Action"=enum."Stop", "Data"=variant}) -> ()  [unwired: 2 in, 3 out]
            n143 = call "HardwareAbortGlobal.vi"("Action"=HardwareAbortGlobalAction."Set", "Set Value"=TRUE) -> ()  [unwired: 9 in, 1 out]
          }
          frame "Hardware Stopped" {
            w188 = T31."Enabled" ("Disabled")
            n144 = local write "Hardware Running?"(FALSE ("Hardware Armed?")) -> ()
            n145 = Enqueue Element(queue=w193, element=T32 {"Action"=enum."Log Stop", "Data"=variant}, error in (no error)=w192) -> (error out=w191:errorcluster)  [unwired: 1 in, 2 out]
            n146 = property on="LOG START" class="Bool (strict)"("DisabledEnum"=T31."Disabled and Grayed Out" ("Disabled")) -> ()  [unwired: 2 in, 2 out]
            n147 = property on="SHOW DUT DIALOG" class="Bool"("DisabledEnum"=w188) -> ()  [unwired: 2 in, 2 out]
            n148 = property on="SHOW LOG DIALOG" class="Bool"("DisabledEnum"=w188) -> ()  [unwired: 2 in, 2 out]
            n149 = property on="SHOW MEASURE DIALOG" class="Bool"("DisabledEnum"=w188) -> ()  [unwired: 2 in, 2 out]
            n150 = property on="SHOW SOURCE DIALOG" class="Bool"("DisabledEnum"=w188) -> ()  [unwired: 2 in, 2 out]
            n151 = property on="SHOW TRIGGER DIALOG" class="Bool"("DisabledEnum"=w188) -> ()  [unwired: 2 in, 2 out]
            n152 = property on="OPEN" class="Bool"("DisabledEnum"=w188) -> ()  [unwired: 2 in, 2 out]
            n153 = property on="RESET" class="Bool"("DisabledEnum"=w188) -> ()  [unwired: 2 in, 2 out]
            n154 = property on="SAVE" class="Bool"("DisabledEnum"=w188) -> ()  [unwired: 2 in, 2 out]
          }
          frame "Log Start" {
            n155 = Flush Queue(queue=w199) -> (queue out=w198:refnum<queue>)  [unwired: 1 in, 2 out]
            n156 = To Variant(anything=w197) -> (Variant=w200:variant)
            n157 = Bundle By Name(cluster=T37 {"Action"=enum."Create", "Data"=variant} ("element"), "Data"=w200) -> (w201:T37)
            n158 = Enqueue Element(queue=w198, element=w201) -> ()  [unwired: 2 in, 3 out]
          }
          frame "Log Arm" {
            n159 = Flush Queue(queue=w207) -> (queue out=w208:refnum<queue>)  [unwired: 1 in, 2 out]
            n160 = To Variant(anything=w206) -> (Variant=w209:variant)
            n161 = Bundle By Name(cluster=T37 {"Action"=enum."Start", "Data"=variant} ("element"), "Data"=w209) -> (w210:T37)
            n162 = Enqueue Element(queue=w208, element=w210) -> ()  [unwired: 2 in, 3 out]
          }
          frame "Log Started" {
            w213 = TRUE ("Log Running?")
            n163 = Variant To Data(type=path "", Variant=w219) -> (data=→"Log File":path)  [unwired: 1 in, 1 out]
            n164 = Unbundle By Name(w214) -> ("Log.Stop.Trigger Type"=w216:T17)
            n165 = case shown="\"File Size\"" w216 {
              tunnel: [T31."Disabled and Grayed Out" ("Disabled") T31."Enabled" ("Disabled") T31."Enabled" ("Disabled") T31."Enabled" ("Disabled") T31."Enabled" ("Disabled")] -> w215
              frame "None", Default {
              }
              frame "User" {
              }
              frame "Timer" {
              }
              frame "File Size" {
              }
              frame "Digital IO" {
              }
            }
            n166 = local write "LOG START"(w213) -> ()
            n167 = property on="LOG START" class="Bool (strict)"("DisabledEnum"=w215) -> ()  [unwired: 2 in, 2 out]
            "Log Running?" <- w213
          }
          frame "Log Stop" {
            n168 = Flush Queue(queue=w230) -> (queue out=w229:refnum<queue>, error out=w228:errorcluster)  [unwired: 1 in, 1 out]
            n169 = Enqueue Element(queue=w229, element=T37 {"Action"=enum."Stop", "Data"=variant}, error in (no error)=w228) -> ()  [unwired: 1 in, 3 out]
          }
          frame "Log Stopped" {
            w238 = FALSE ("Log Running?")
            n170 = Unbundle By Name(w237) -> ("Log"=w236:T10)
            n171 = Unbundle By Name(w236) -> ("Start.Trigger Type"=w235:T12)
            n172 = case shown="\"User\"" w235 {
              tunnel: [T31."Disabled and Grayed Out" ("Disabled") w243 T31."Disabled and Grayed Out" ("Disabled") T31."Disabled and Grayed Out" ("Disabled")] -> w234
              frame "Immediate", Default {
              }
              frame "User" {
                n173 = local read "Hardware Running?"() -> (w246:bool)
                n174 = Select(t=T31."Enabled" ("Disabled"), s=w246, f=T31."Disabled and Grayed Out") -> (s? t:f=w243:T31)
              }
              frame "Timer" {
              }
              frame "Digital IO" {
              }
            }
            n175 = local write "Log Running?"(w238) -> ()
            n176 = local write "LOG START"(w238) -> ()
            n177 = local write "Log File"(path "") -> ()
            n178 = property on="LOG START" class="Bool (strict)"("DisabledEnum"=w234) -> ()  [unwired: 2 in, 2 out]
          }
          frame "Error" {
            n179 = Variant To Data(type=w250, Variant=w251) -> (data=w249:errorcluster)  [unwired: 1 in, 1 out]
            n180 = call <vilib>:"General Error Handler.vi"("error in (no error)"=w249) -> ()  [unwired: 10 in, 5 out]
          }
          frame "Shutdown" {
            n181 = Release Queue(queue=w265, error in (no error)=w264) -> (error out=w263:errorcluster)  [unwired: 1 in, 2 out]
            n182 = Flush Queue(queue=w262) -> (queue out=w256:refnum<queue>)  [unwired: 1 in, 2 out]
            n183 = Flush Queue(queue=w259) -> (queue out=w258:refnum<queue>)  [unwired: 1 in, 2 out]
            n184 = Not(x=w267) -> (.not. x?=w266:bool)
            n185 = local read "Hardware START"() -> (w255:bool)
            n186 = Enqueue Element(queue=w258, element=T37 {"Action"=enum."Shutdown", "Data"=variant}) -> ()  [unwired: 2 in, 3 out]
            n187 = case shown="True" w255 {
              tunnel: w256 -> [w268 w270]
              tunnel: [w268 w269] -> w254
              frame False {
              }
              frame True {
                n188 = Enqueue Element(queue=w270, element=T34 {"Action"=enum."Stop", "Data"=variant}) -> (queue out=w269:refnum<queue>)  [unwired: 2 in, 2 out]
              }
            }
            n189 = Enqueue Element(queue=w254, element=T34 {"Action"=enum."Shutdown", "Data"=variant}) -> ()  [unwired: 2 in, 3 out]
          }
        }
      }
      n190 = Merge Errors(w29, w26) -> (w28:errorcluster)
    }
    frame Error {
    }
  }
  n191 = call "HardwareLoop.vi"("Error In"=w7, "Executable Configuration"=w2, "Data Structures"=w5, "Action Queues"=w6) -> ("Error Out"=w12:errorcluster)  [unwired: 7 in]
  n192 = call "LogLoop.vi"("Error In"=w7, "Executable Configuration"=w2, "Data Structures"=w5, "Action Queues"=w6) -> ("Error Out"=w4:errorcluster)  [unwired: 7 in]
  n193 = Merge Errors(w14, w12, w4) -> (w13:errorcluster)
  n194 = call "Shutdown.vi"("Error In"=w13) -> ()  [unwired: 10 in, 1 out]
